vi "Material-Automation-LaunchConfigDialog.vi"(11 "error in":errorcluster) -> (15 "error out":errorcluster)   [LabVIEW 2013]
panel:
  # "Inputs"
  # "Outputs"
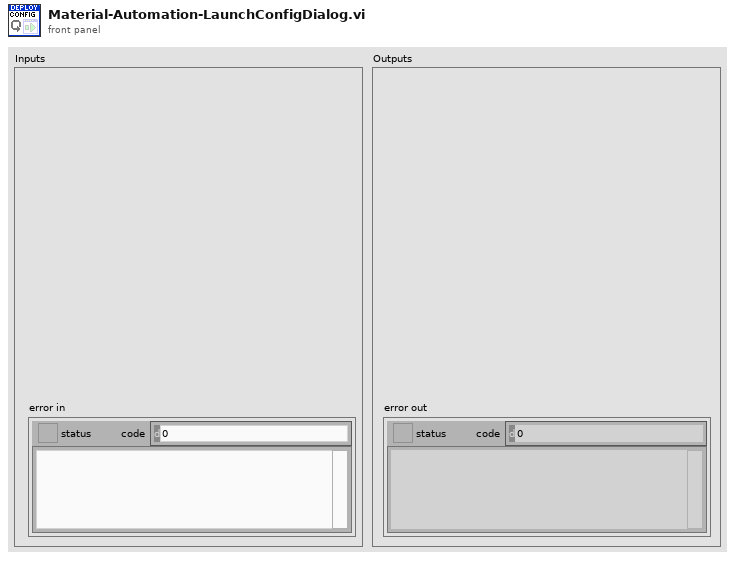
[diagram p1: front panel]
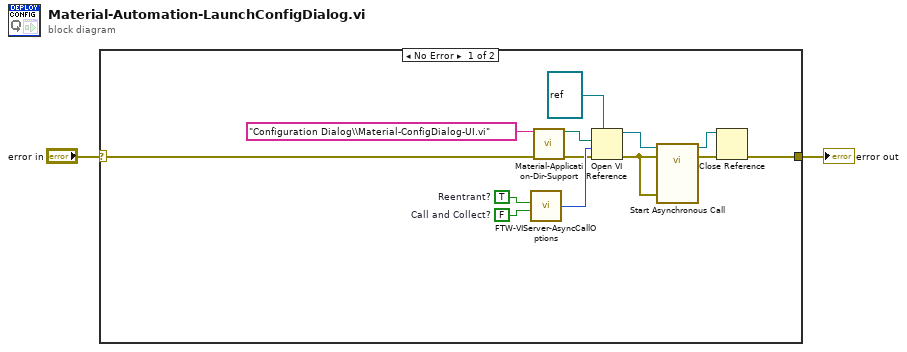
[diagram p0: block diagram]
diagram:
  n1 = case shown="No Error" "error in" {
    selector: "error in" -> [w11 w16]
    tunnel: [w15 w16] -> w2
    frame No Error {
      w12 = FALSE  # Call and Collect?
      w13 = TRUE  # Reentrant?
      n2 = call "FTW-VIServer-AsyncCallOptions.vi"("Call and Collect?"=w12, "Reentrant?"=w13) -> ("Open VI Ref Options"=w14:i32)  [unwired: 4 in]
      n3 = call "Material-Application-Dir-Support.vi"("Support Resource Relative Filepath"="Configuration Dialog\\Material-ConfigDialog-UI.vi" ("Support VI Relative Filepath"), "error in"=w11) -> ("Support Filepath"=w9:path, "error out"=w10:errorcluster)  [unwired: 12 in]
      n4 = Open VI Reference(type specifier VI Refnum (for type only)=refnum<vi> refnum, vi path=w9, options=w14, error in (no error)=w10) -> (vi reference=w8:refnum<vi>, error out=w4:errorcluster)  [unwired: 2 in]
      n5 = call-by-ref "Start Asynchronous Call"(reference=w8, error in=w4, "error in"=w4) -> (reference out=w5:refnum<vi>, error out=w6:errorcluster)  [unwired: 14 in, 1 out]
      n6 = Close Reference(reference=w5, error in (no error)=w6) -> (error out=w15:errorcluster)
    }
    frame Error {
    }
  }
  "error out" <- w2
